vi "Read Piezo Main.vi"(0 "object in":refnum<class "TBS2000Series.lvclass">, 5 "error in (no error)":errorcluster) -> (14 "object out":refnum<class "TBS2000Series.lvclass">, 15 "Frequency":dbl format="%.2p", 16 "Peak-to-Peak":dbl format="%.2p", 17 "Main Channel":T1(graph), 19 "error out":errorcluster)   [LabVIEW 2023, in "TBS2000Series.lvclass"]
uses:
  TBS2000Series.lvclass
  TBS2000Series.lvclass/TBS2000Series.ctl
  <instrlib>/Tektronix TBS 2000 Series/Tektronix TBS 2000 Series.lvlib
panel:
  in  "Timebase (4.00 us) 3":dbl=4e-06 format="%.2p"
  in  "Timebase (4.00 us) 2":dbl=4e-06 format="%.2p"
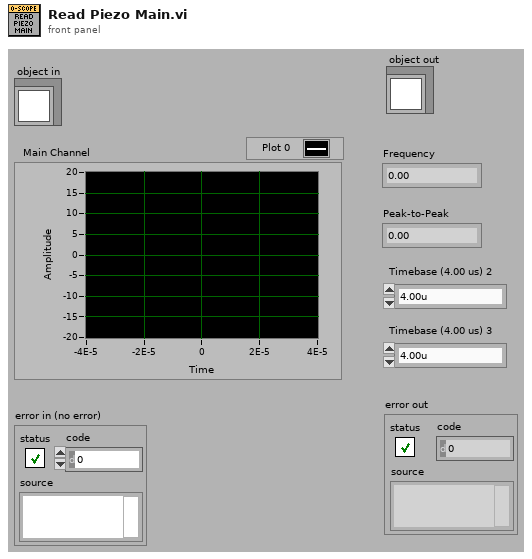
[diagram p1: front panel]
types:
  T1 = cluster{"Initial X":dbl, "X Increment":dbl, "Waveform Array":dbl[]}
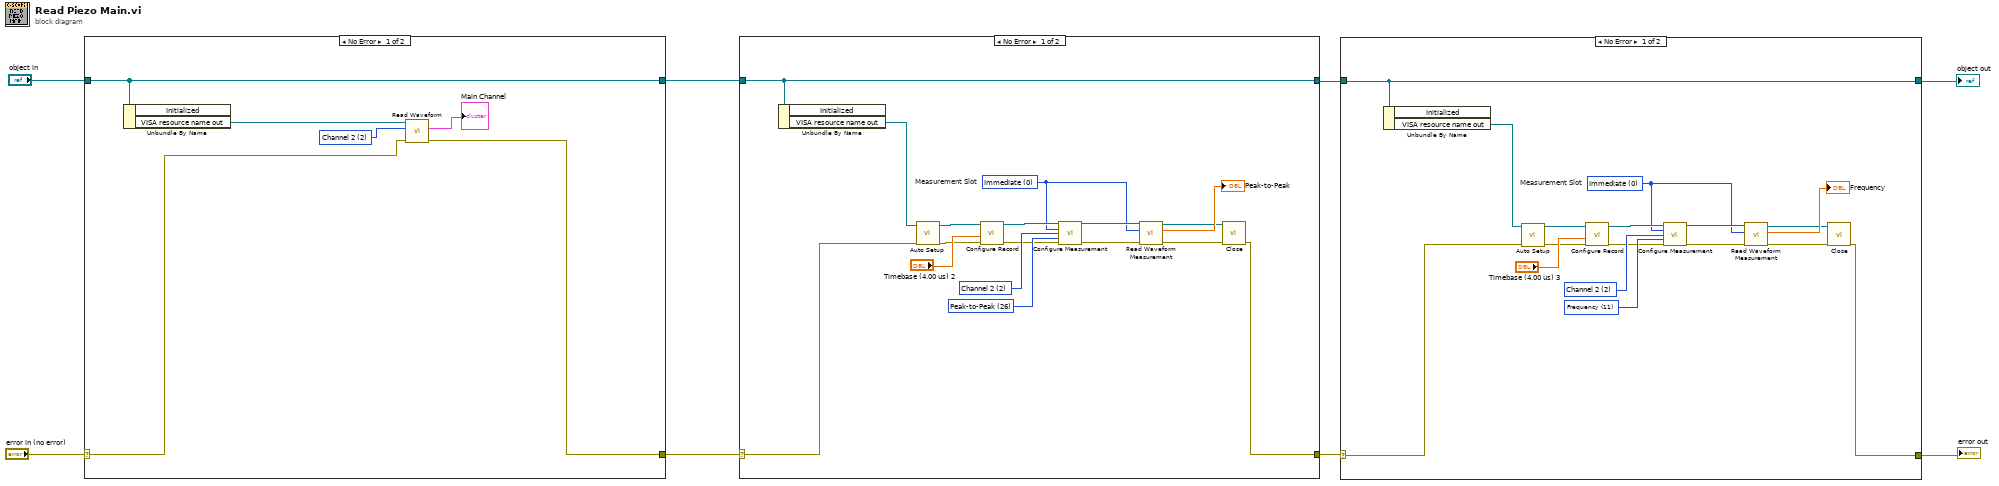
[diagram p0: block diagram]
diagram:
  n1 = case shown="No Error" "error in (no error)" {
    selector: "error in (no error)" -> [w10 w16]
    tunnel: [w9 w16] -> w4
    tunnel: [w14 w15] -> w1
    tunnel: "object in" -> [w14 w15]
    frame No Error {
      w13 = 2 items=["Math", "Channel 1", "Channel 2", "Channel 3", "Channel 4"] ("Source (1: Channel 1)")
      n2 = Unbundle By Name(w14) -> ("VISA resource name out"=w11:refnum<visa-resource-name>)  [unwired: 1 out]
      n3 = call <instrlib>:"Read Waveform.vi"("error in (no error)"=w10, "Source (1: Channel 1)"=w13, "VISA resource name"=w11) -> ("error out"=w9:errorcluster, "Waveform Graph"=→"Main Channel":T1)  [unwired: 6 in, 1 out]
    }
    frame Error {
    }
  }
  n4 = case shown="No Error" w4 {
    selector: w4 -> [w19 w35]
    tunnel: [w17 w35] -> w6
    tunnel: [w33 w34] -> w2
    tunnel: w1 -> [w33 w34]
    frame No Error {
      w31 = 26 items=["Amplitude", "Area", "Burst", "Cycle Area", "Cycle Mean", "Cycle RMS", "Delay RR", "Delay RF", "Delay FR", "Delay FF", "Fall Time", "Frequency", "High Reference", "Low Reference", "Max", "Mean", "Min", "- Duty Cycle", "- Edge Count", "- Overshoot", "- Pulse Count", "- Width", "+ Duty Cycle", "+ Edge Count", "Period", "Phase", "Peak-to-Peak", "+ Overshoot", "+ Pulse Count", "+ Width", "Rise", "RMS"] ("Measurement Type (0: Amplitude)")
      w30 = 2 items=["Math", "Channel 1", "Channel 2", "Channel 3", "Channel 4"] ("Measurement Source 1 (1: Channel 1)")
      w25 = 0 items=["Immediate", "Measurement 1", "Measurement 2", "Measurement 3", "Measurement 4", "Measurement 5", "Measurement 6"]  # Measurement Slot
      n5 = Unbundle By Name(w33) -> ("VISA resource name out"=w22:refnum<visa-resource-name>)  [unwired: 1 out]
      n6 = call <instrlib>:"Auto Setup.vi"("error in (no error)"=w19, "VISA resource name"=w22) -> ("error out"=w20:errorcluster, "VISA resource name out"=w21:refnum<visa-resource-name>)  [unwired: 8 in]
      n7 = call <instrlib>:"Configure Record.vi"("error in (no error)"=w20, "Timebase (4.00 us)"="Timebase (4.00 us) 2", "VISA resource name"=w21) -> ("error out"=w18:errorcluster, "VISA resource name out"=w26:refnum<visa-resource-name>)  [unwired: 7 in]
      n8 = call <instrlib>:"Configure Measurement.vi"("VISA resource name"=w26, "Measurement Slot (0: Immediate)"=w25, "Measurement Source 1 (1: Channel 1)"=w30, "Measurement Type (30: Rise)"=w31, "error in (no error)"=w18) -> ("VISA resource name out"=w28:refnum<visa-resource-name>, "error out"=w27:errorcluster)  [unwired: 9 in]
      n9 = call <instrlib>:"Read Waveform Measurement.vi"("error in (no error)"=w27, "Measurement Slot (0: Immediate)"=w25, "VISA resource name"=w28) -> ("error out"=w23:errorcluster, "Measurement"=→"Peak-to-Peak":dbl, "VISA resource name out"=w24:refnum<visa-resource-name>)  [unwired: 6 in]
      n10 = call <instrlib>:"Close.vi"("error in (no error)"=w23, "VISA resource name"=w24) -> ("error out"=w17:errorcluster)  [unwired: 9 in]
    }
    frame Error {
    }
  }
  n11 = case shown="No Error" w6 {
    selector: w6 -> [w37 w54]
    tunnel: [w36 w54] -> w5
    tunnel: [w38 w53] -> w3
    tunnel: w2 -> [w38 w53]
    frame No Error {
      w51 = 11 items=["Amplitude", "Area", "Burst", "Cycle Area", "Cycle Mean", "Cycle RMS", "Delay RR", "Delay RF", "Delay FR", "Delay FF", "Fall Time", "Frequency", "High Reference", "Low Reference", "Max", "Mean", "Min", "- Duty Cycle", "- Edge Count", "- Overshoot", "- Pulse Count", "- Width", "+ Duty Cycle", "+ Edge Count", "Period", "Phase", "Peak-to-Peak", "+ Overshoot", "+ Pulse Count", "+ Width", "Rise", "RMS"] ("Measurement Type (0: Amplitude)")
      w50 = 2 items=["Math", "Channel 1", "Channel 2", "Channel 3", "Channel 4"] ("Measurement Source 1 (1: Channel 1)")
      w45 = 0 items=["Immediate", "Measurement 1", "Measurement 2", "Measurement 3", "Measurement 4", "Measurement 5", "Measurement 6"]  # Measurement Slot
      n12 = Unbundle By Name(w38) -> ("VISA resource name out"=w42:refnum<visa-resource-name>)  [unwired: 1 out]
      n13 = call <instrlib>:"Auto Setup.vi"("error in (no error)"=w37, "VISA resource name"=w42) -> ("error out"=w40:errorcluster, "VISA resource name out"=w41:refnum<visa-resource-name>)  [unwired: 8 in]
      n14 = call <instrlib>:"Configure Record.vi"("error in (no error)"=w40, "Timebase (4.00 us)"="Timebase (4.00 us) 3", "VISA resource name"=w41) -> ("error out"=w39:errorcluster, "VISA resource name out"=w46:refnum<visa-resource-name>)  [unwired: 7 in]
      n15 = call <instrlib>:"Configure Measurement.vi"("VISA resource name"=w46, "Measurement Slot (0: Immediate)"=w45, "Measurement Source 1 (1: Channel 1)"=w50, "Measurement Type (30: Rise)"=w51, "error in (no error)"=w39) -> ("VISA resource name out"=w48:refnum<visa-resource-name>, "error out"=w47:errorcluster)  [unwired: 9 in]
      n16 = call <instrlib>:"Read Waveform Measurement.vi"("error in (no error)"=w47, "Measurement Slot (0: Immediate)"=w45, "VISA resource name"=w48) -> ("error out"=w43:errorcluster, "Measurement"=→"Frequency":dbl, "VISA resource name out"=w44:refnum<visa-resource-name>)  [unwired: 6 in]
      n17 = call <instrlib>:"Close.vi"("error in (no error)"=w43, "VISA resource name"=w44) -> ("error out"=w36:errorcluster)  [unwired: 9 in]
    }
    frame Error {
    }
  }
  "error out" <- w5
  "object out" <- w3
